vi "Configure Limit.vi"(7 "Enable Limit (F: Disable)":bool, 8 "error in (no error)":errorcluster, 9 "Upper Limit (0)":dbl, 10 "Lower Limit (0)":dbl, 11 "VISA resource name":refnum<visa-resource-name>) -> (0 "error out":errorcluster, 3 "VISA resource name out":refnum<visa-resource-name>)   [LabVIEW 2013, in "Agilent 3446X Series.lvlib"]
doc: "Configures the settings of limit testing."
uses:
  <instrlib>/Agilent 3446X Series/Agilent 3446X Series.lvlib
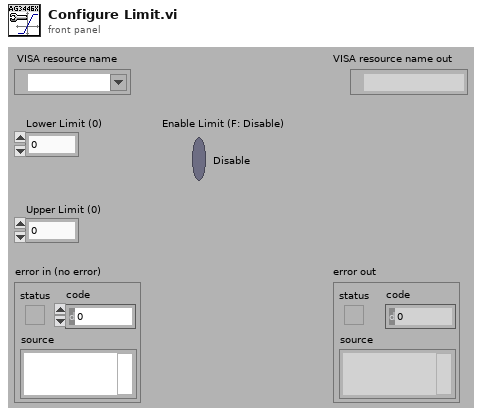
[diagram p1: front panel]
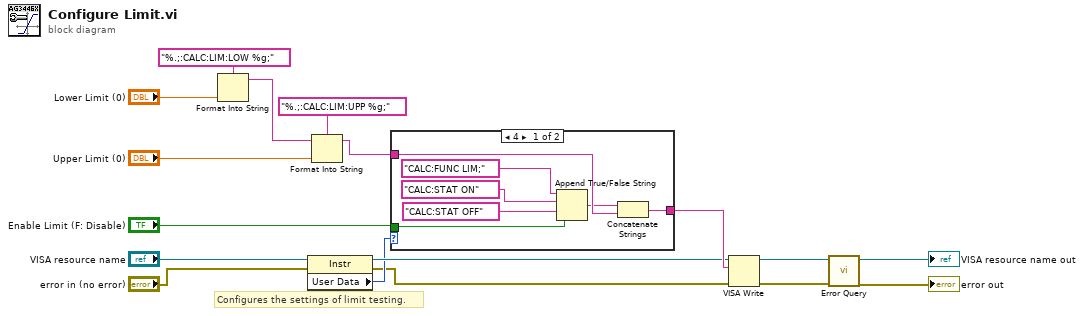
[diagram p0: block diagram]
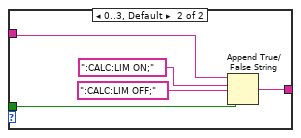
[diagram p2: hidden frame]
diagram:
  # "Configures the settings of limit testing."
  n1 = Format Into String(format string="%.;:CALC:LIM:LOW %g;", "Lower Limit (0)") -> (resulting string=w3:string)  [unwired: 2 in, 1 out]
  n2 = property class="Instr"(reference="VISA resource name", error in="error in (no error)") -> (reference out=w7:refnum<visa-resource-name>, error out=w4:errorcluster, "User Data"=w6:u32)
  n3 = Format Into String(format string="%.;:CALC:LIM:UPP %g;", initial string=w3, "Upper Limit (0)") -> (resulting string=w9:string)  [unwired: 1 in, 1 out]
  n4 = case shown="4" w6 {
    tunnel: [w18 w28] -> w14
    tunnel: w9 -> [w20 w27]
    tunnel: "Enable Limit (F: Disable)" -> [w22 w25]
    frame 4 {
      n5 = Append True/False String(1:w22, 2:"CALC:STAT OFF" ("false string"), 3:"CALC:STAT ON" ("true string"), 4:"CALC:FUNC LIM;" ("string")) -> (0:w19:string)
      n6 = Concatenate Strings(w19, w20) -> (w18:string)
    }
    frame 0..3, Default {
      n7 = Append True/False String(1:w25, 2:":CALC:LIM OFF;", 3:":CALC:LIM ON;" ("true string"), 4:w27) -> (0:w28:string)
    }
  }
  n8 = VISA Write(VISA resource name=w7, write buffer=w14, error in (no error)=w4) -> (VISA resource name out=w13:refnum<visa-resource-name>, error out=w12:errorcluster)  [unwired: 1 out]
  n9 = call <instrlib>:"Error Query.vi"("error in (no error)"=w12, "VISA resource name"=w13) -> ("error out"=→"error out":errorcluster, "VISA resource name out"=→"VISA resource name out":refnum<visa-resource-name>)  [unwired: 8 out]
